vi "Wait for TCP Ack.vi"(6 "options":T3={"ignore timeout error"=TRUE, "timeout ms (1000)"=1000}, 8 "error in (no error)":errorcluster, 10 "cmd name":string, 11 "connection info in":T1) -> (0 "error out":errorcluster, 2 "timeout":bool, 3 "connection info out":T1)   [LabVIEW 2021, in "AudioGeneration.lvclass"]
uses:
  AudioGeneration.lvclass
  <vilib>/NI/STM/TCP/TCP Write Options.ctl
  <vilib>/NI/STM/TCP/TCP Connection Info.ctl
  <vilib>/NI/STM/SubVIs/MetaDataElement.ctl
  <vilib>/NI/STM/TCP/Read Message (TCP).vi
  <vilib>/NI/STM/NI STM.lvlib
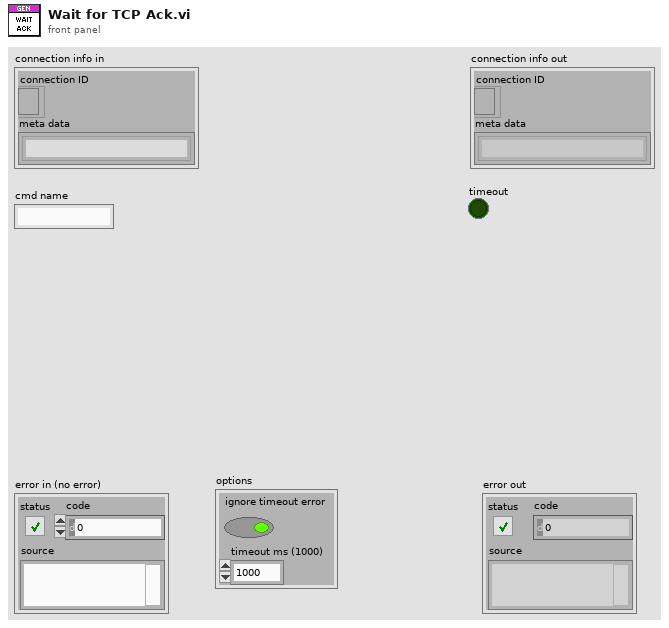
[diagram p1: front panel]
types:
  T1 = typedef "NI STM.lvlib/TCP Connection Info.ctl" = cluster{"connection ID":refnum<k5>, "meta data":T2[]}
  T2 = typedef "NI STM.lvlib/MetaDataElement.ctl" = string
  T3 = typedef "NI STM.lvlib/TCP Write Options.ctl" = cluster{"ignore timeout error":bool, "timeout ms (1000)":i32}
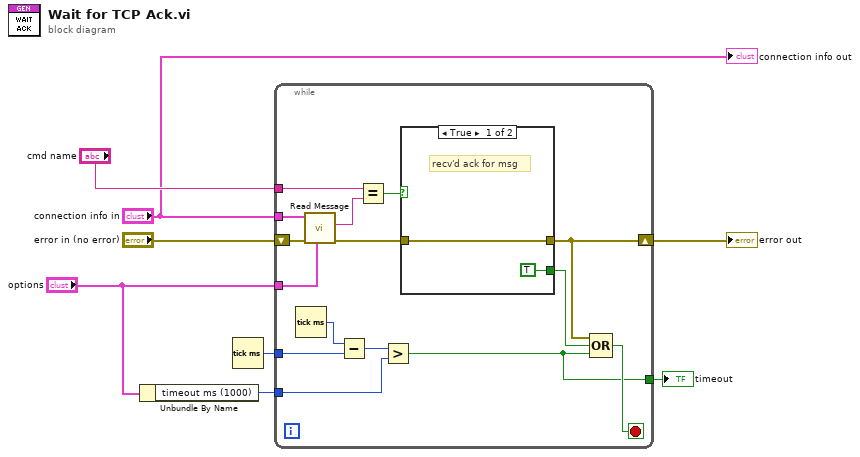
[diagram p0: block diagram]
diagram:
  n1 = Unbundle By Name("options") -> ("timeout ms (1000)"=w7:i32)
  n2 = Tick Count (ms)() -> (millisecond timer value=w5:u32)
  n3 = while {
    tunnel: "connection info in" -> [w22]
    tunnel: "cmd name" -> [w20]
    tunnel: "options" -> [w10]
    shift-right: [w14] -> w3
    shift-left: "error in (no error)" -> [w23]
    tunnel: w5 -> [w16]
    tunnel: w7 -> [w11]
    tunnel: [w9] -> w8
    stop <- w12 stop-if-true
    n4 = Tick Count (ms)() -> (millisecond timer value=w17:u32)
    n5 = call-poly <vilib>:"Read Message.vi"("options"=w10, "error in"=w23, "connection info in"=w22) -> ("error out"=w21:errorcluster, "data string"=w19:string)  [unwired: 3 in, 4 out]
    n6 = Subtract(x=w17, y=w16) -> (x-y=w15:u32)
    n7 = Equal?(x=w20, y=w19) -> (x = y?=w18:bool)
    n8 = Greater?(x=w15, y=w11) -> (0:w9:bool)
    n9 = case shown="True" w18 {
      tunnel: w21 -> [w25 _]
      tunnel: [w25 _] -> w14
      tunnel: [TRUE _] -> w13
      frame True {
        # "recv'd ack for msg"
      }
      frame False {
      }
    }
    n10 = Compound Arithmetic op=OR(w14, w13, w9) -> (w12:bool)
  }
  "timeout" <- w8
  "error out" <- w3
  "connection info out" <- "connection info in"
